vi "WT300 Reset and Clear Errors.vi"(8 "error in (no error)":errorcluster, 11 "VISA Refnum in":refnum<visa-resource-name>) -> (0 "error out":errorcluster, 3 "VISA Refnum out":refnum<visa-resource-name>)   [LabVIEW 2023]
uses:
  Yokogawa WT300 Series.lvlib
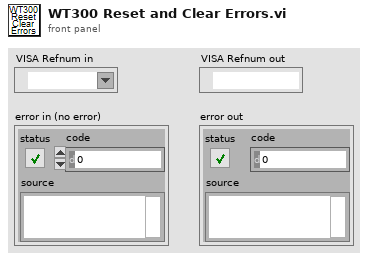
[diagram p1: front panel]
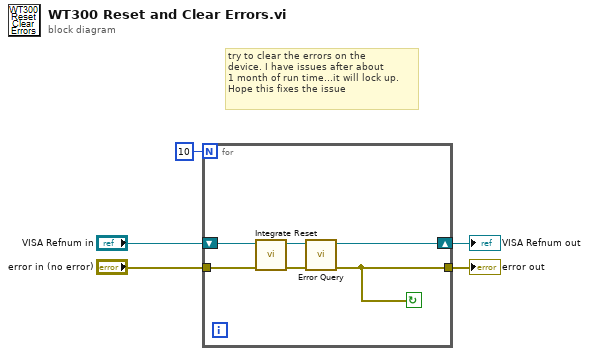
[diagram p0: block diagram]
diagram:
  # "try to clear the errors on the \ndevice. I have issues after about\n1 month of run time...it will lock up.\nHope this fixes the issue"
  n1 = for {
    N: 10 -> [_]
    shift-right: [w7] -> w3
    shift-left: "VISA Refnum in" -> [w11]
    tunnel: "error in (no error)" -> [w10]
    tunnel: [w6] -> w4
    stop <- w6 continue-if-true
    n2 = call "Integrate Reset.vi"("error in (no error)"=w10, "VISA resource name"=w11) -> ("error out"=w9:errorcluster, "VISA resource name out"=w8:refnum<visa-resource-name>)  [unwired: 8 in]
    n3 = call "Error Query.vi"("error in (no error)"=w9, "VISA resource name"=w8) -> ("error out"=w6:errorcluster, "VISA resource name out"=w7:refnum<visa-resource-name>)  [unwired: 6 in, 2 out]
  }
  "error out" <- w4
  "VISA Refnum out" <- w3
